vi "Do.vi"(8 "error in (no error)":errorcluster, 10 "Actor in":refnum<class "Actor.lvclass">, 11 "New Camera Settings Msg":refnum<class "New Camera Settings Msg.lvclass">) -> (0 "error out":errorcluster, 2 "Actor out":refnum<class "Actor.lvclass">)   [LabVIEW 2020, in "New Camera Settings Msg.lvclass"]
doc: "This VI delivers the message to the actor by calling the appropriate method(s) on the actor."
uses:
  New Camera Settings Msg.lvclass
  C:/Users/AlexK/work/LabVIEW Programme/POLARIS-AS-3-Cams/Submodules/HIJ Vision/Camera Actors/Camera Actor/Camera Actor Messages/Publish Camera Settings Msg/Publish Camera Settings Msg.lvclass
  <vilib>/ActorFramework/Actor/Actor.lvclass
  HIJ Vision Camera App/HIJ Vision Camera App.lvclass
  C:/Program Files (x86)/National Instruments/LabVIEW 2020/vi.lib/ActorFramework/Actor/Actor.lvclass
  Camera Actors/Camera Actor/Camera Actor Messages/Publish Camera Settings Msg/Publish Camera Settings Msg.lvclass
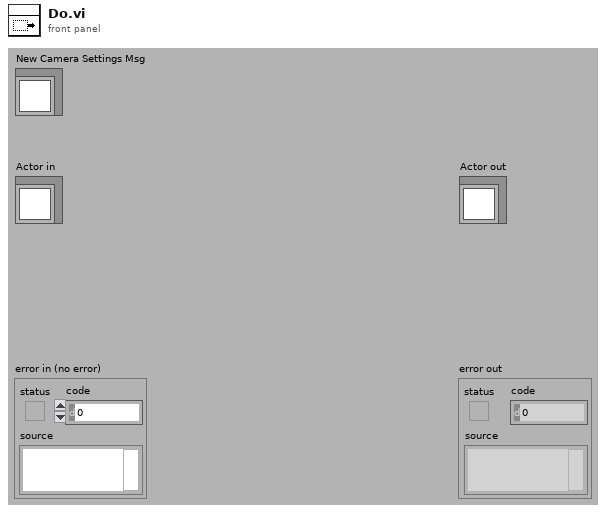
[diagram p1: front panel]
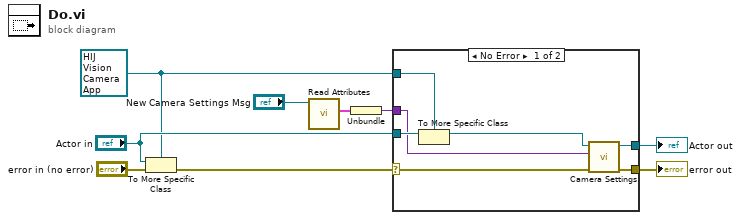
[diagram p0: block diagram]
diagram:
  w4 = refnum<class "HIJ Vision Camera App.lvclass"> refnum ("Actor in")
  n1 = To More Specific Class(target class=w4, reference="Actor in", error in="error in (no error)") -> (error out=w8:errorcluster)  [unwired: 1 out]
  n2 = call "Read Attributes.vi"("Abstract Message Template in"="New Camera Settings Msg") -> ("Payload"=w2:cluster{"Camera Settings":variant})  [unwired: 9 in, 1 out]
  n3 = Unbundle(w2) -> ("Camera Settings"=w1:variant)
  n4 = case shown="No Error" w8 {
    selector: w8 -> [w14 w18]
    tunnel: [w16 w18] -> w7
    tunnel: [w15 w17] -> w6
    tunnel: "Actor in" -> [w13 w17]
    tunnel: w4 -> [w12 _]
    tunnel: w1 -> [w11 _]
    frame No Error {
      n5 = To More Specific Class(target class=w12, reference=w13) -> (specific class reference=w10:refnum<class "HIJ Vision Camera App.lvclass">)  [unwired: 1 in, 1 out]
      n6 = call-dynamic "Camera Settings.vi"("error in (no error)"=w14, "Camera Settings"=w11, "HIJ Vision Camera App in"=w10) -> ("error out"=w16:errorcluster, "HIJ Vision Camera App out"=w15:refnum<class "HIJ Vision Camera App.lvclass">)  [unwired: 7 in]
    }
    frame Error {
      # "If type check fails, pass the original object out again."
    }
  }
  "error out" <- w7
  "Actor out" <- w6
